vi "Get Single Control.vi"(8 "error in (no error)":errorcluster, 10 "Control Name":string, 11 "Controls_Mgr in":refnum<class "Controls_Mgr.lvclass">) -> (0 "error out":errorcluster, 2 "Variant":variant, 3 "Controls_Mgr out":refnum<class "Controls_Mgr.lvclass">)   [LabVIEW 2015, in "Generic Module Library.lvlib" / "Template G_Module.lvlib" / "Controls_Mgr.lvclass"]
uses:
  Controls_Mgr.lvclass
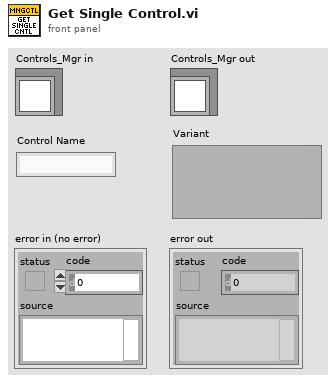
[diagram p1: front panel]
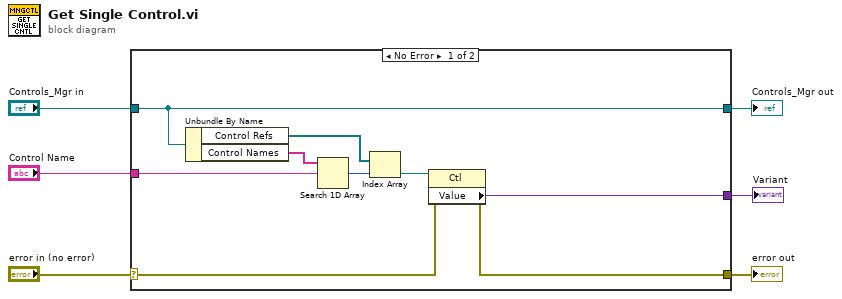
[diagram p0: block diagram]
diagram:
  n1 = case shown="No Error" "error in (no error)" {
    selector: "error in (no error)" -> [w9 w17]
    tunnel: [w8 w17] -> w5
    tunnel: [w12 w16] -> w3
    tunnel: "Controls_Mgr in" -> [w12 w16]
    tunnel: "Control Name" -> [w11 _]
    tunnel: [w7 _] -> w1
    frame No Error {
      n2 = Unbundle By Name(w12) -> ("Control Refs"=w13:refnum<vi>[], "Control Names"=w15:string[])
      n3 = Search 1D Array(1D array=w15, element=w11) -> (index of element=w14:i32)  [unwired: 1 in]
      n4 = Index Array(array=w13, index=w14) -> (element=w10:refnum<vi>)
      n5 = property class="Ctl"(reference=w10, error in=w9) -> (error out=w8:errorcluster, "Value"=w7:variant)  [unwired: 1 out]
    }
    frame Error {
    }
  }
  "error out" <- w5
  "Controls_Mgr out" <- w3
  "Variant" <- w1
